vi "CVT1IndexWriteTest.vi"() -> (3 "Unit Test Framework Results":T1)   [LabVIEW 2013, in "UnitTests.lvlib"]
uses:
  UnitTests.lvlib
  <vilib>/utf/common/utf_test_result_troll.ctl
  <vilib>/utf/common/utf_test_result.ctl
  <vilib>/utf/common/utf_test_result_failure.ctl
  <vilib>/utf/common/utf_test_comparison_operators.ctl
  <vilib>/utf/common/utf_vi_tag.ctl
  <vilib>/NI/Current Value Table/Write Index.vi
  <vilib>/NI/Current Value Table/DataTypes/I32_Write Index.vi
  <vilib>/NI/Current Value Table/Read Index.vi
  <vilib>/NI/Current Value Table/DataTypes/I32_Read Index.vi
  <vilib>/NI/Current Value Table/Compatibility/TagConverter.vi
  <vilib>/NI/Current Value Table/Create Tags.vi
  <vilib>/NI/Current Value Table/Memory Block.vi
  <vilib>/NI/Current Value Table/DataTypes/I32_Memory Block.vi
  <vilib>/utf/NI_UnitTestFramework.lvlib
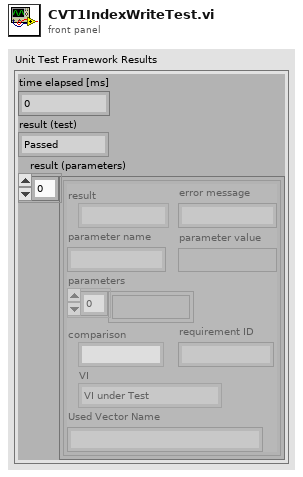
[diagram p1: front panel]
types:
  T1 = typedef "NI_UnitTestFramework.lvlib/utf_test_result_troll.ctl" = cluster{"time elapsed [ms]":u32, "result (test)":T2, "result (parameters)":T3[]}
  T2 = typedef "NI_UnitTestFramework.lvlib/utf_test_result.ctl" = enum16{"Passed", "Failed", "Error", "Skipped", "Not Processed"}
  T3 = typedef "NI_UnitTestFramework.lvlib/utf_test_result_failure.ctl" = cluster{"result":T2, "error message":string, "parameter name":string, "parameter value":variant, "parameters":variant[], "comparison":T4, "requirement ID":string, "VI":T5, "Used Vector Name":string}
  T4 = typedef "NI_UnitTestFramework.lvlib/utf_test_comparison_operators.ctl" = enum16{"=", "!=", ">", ">=", "<", "<=", "range", "symmetric tolerance", "asymmetric tolerance", "string contains", "string not contain", "array size", "string length", "array range", "by element", "array range (limit array)", "user-defined", "array contains", "array not contain", "vector length", "= (elm)", "!= (elm)", "= (case insensitive)", "!= (case insensitive)"}
  T5 = typedef "NI_UnitTestFramework.lvlib/utf_vi_tag.ctl" = enum16{"Setup VI", "VI under Test", "Teardown VI"}
  T6 = typedef "cvt_Tag Configuration.ctl" = cluster{"Name":string, "Data Type":T7, "Array":bool, "Size":u32, "Default":string, "Enum":string[], "Description":string}
  T7 = typedef "cvt_Data Types.ctl" = enum16{"Bool", "U8", "I32", "Double", "String", "Enum"}
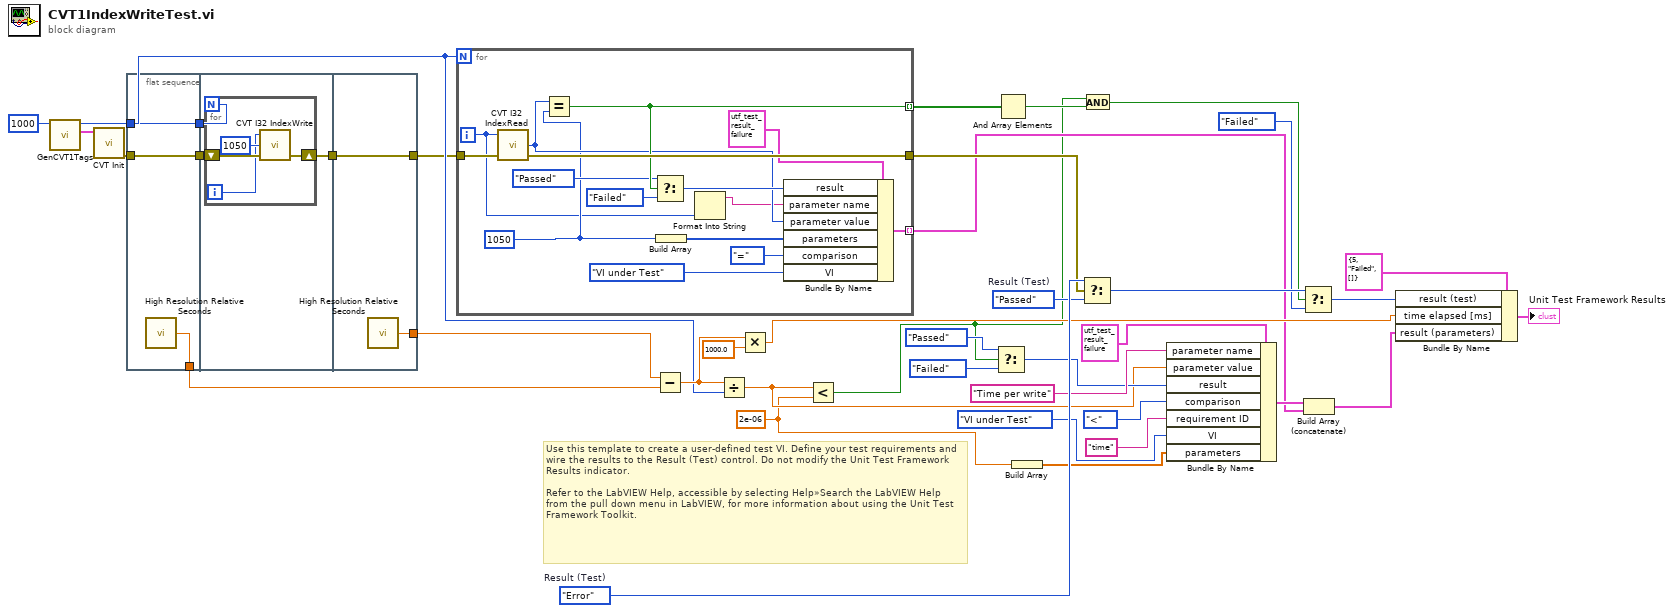
[diagram p0: block diagram]
diagram:
  w5 = 2e-06 ("y")
  w34 = utf_test_result."Error"  # Result (Test)
  w33 = utf_test_result."Passed"  # Result (Test)
  # "Use this template to create a user-defined test VI. Define your test requirements and wire the results to the Result (Test) control. Do not modify the Unit Test Framework Results indicator. \n\nRefer to the LabVIEW Help, accessible by selecting Help»Search the LabVIEW Help from the pull down menu in LabVIEW, for more information about using the Unit Test Framework Toolkit."
  n1 = call "GenCVT1Tags.vi"("Number of Tags in"=1000) -> ("Tags"=w27:T6[], "Number of Tags out"=w20:i32)  [unwired: 8 in, 1 out]
  n2 = call <vilib>:"CVT Init.vi"("Tag List"=w27) -> ("error out"=w26:errorcluster)  [unwired: 10 in]
  n3 = flat-sequence {
    tunnel: [w42] -> w36
    tunnel: w26 -> [w40]
    tunnel: [w41] -> w25
    tunnel: w20 -> [w41]
    tunnel: [w40] -> w24
    tunnel: w25 -> [w45]
    tunnel: w24 -> [w44]
    tunnel: [w43] -> w23
    tunnel: [w51] -> w37
    tunnel: w23 -> [w50]
    tunnel: [w50] -> w19
    frame #0 {
      n4 = call <vilib>:"High Resolution Relative Seconds.vi"() -> ("relative seconds"=w42:dbl)
    }
    frame #1 {
      n5 = for {
        N: w45 -> [_]
        shift-right: [w48] -> w43
        shift-left: w44 -> [w49]
        i -> [w46]
        n6 = call <vilib>:"CVT I32 IndexWrite.vi"("error in (no error)"=w49, "Value"=1050, "Tag Index"=w46) -> ("error out"=w48:errorcluster)  [unwired: 2 in]
      }
    }
    frame #2 {
      n7 = call <vilib>:"High Resolution Relative Seconds.vi"() -> ("relative seconds"=w51:dbl)
    }
  }
  n8 = for {
    N: w20 -> [_]
    tunnel: w19 -> [w66]
    tunnel: [w65] -> w18
    tunnel: [w62] -> w17 mode=indexing
    tunnel: [w58] -> w3 mode=indexing
    i -> [w53]
    w54 = 1050 ("Value")
    n9 = call <vilib>:"CVT I32 IndexRead.vi"("error in (no error)"=w66, "Tag Index"=w53) -> ("error out"=w65:errorcluster, "Value"=w55:i32)  [unwired: 2 in]
    n10 = Equal?(x=w55, y=w54) -> (x = y?=w62:bool)
    n11 = Select(t=utf_test_result."Passed" ("result"), s=w62, f=utf_test_result."Failed" ("result")) -> (s? t:f=w59:T2)
    n12 = Build Array(w54) -> (w56:i32[])
    n13 = Format Into String(w53) -> (resulting string=w52:string)  [unwired: 3 in, 1 out]
    n14 = Bundle By Name(cluster=T3 {"result"=enum."Passed", "error message"="", "parameter name"="", "parameter value"=variant, "parameters"=[], "comparison"=enum."=", "requirement ID"="", "VI"=enum."Setup VI", "Used Vector Name"=""} ("Unit Test Framework - result (parameters)"), "result"=w59, "parameter name"=w52, "parameter value"=w55, "parameters"=w56, "comparison"=utf_test_comparison_operators."=", "VI"=utf_vi_tag."VI under Test") -> (w58:T3)
  }
  n15 = Subtract(x=w37, y=w36) -> (x-y=w22:dbl)
  n16 = Divide(x=w22, y=w20) -> (x/y=w8:dbl)
  n17 = Multiply(x=w22, y=1000.0) -> (x*y=w28:dbl)
  n18 = Less?(x=w8, y=w5) -> (x < y?=w1:bool)
  n19 = Select(t=utf_test_result."Passed" ("result"), s=w1, f=utf_test_result."Failed" ("result")) -> (s? t:f=w9:T2)
  n20 = And Array Elements(Boolean array=w17) -> (logical AND=w16:bool)
  n21 = Build Array(w5) -> (w4:dbl[])
  n22 = Select(t=w34, s=w18, f=w33) -> (s? t:f=w15:T2)
  n23 = And(x=w1, y=w16) -> (x .and. y?=w2:bool)
  n24 = Bundle By Name(cluster=T3 {"result"=enum."Passed", "error message"="", "parameter name"="", "parameter value"=variant, "parameters"=[], "comparison"=enum."=", "requirement ID"="", "VI"=enum."Setup VI", "Used Vector Name"=""} ("Unit Test Framework - result (parameters)"), "parameter name"="Time per write", "parameter value"=w8, "result"=w9, "comparison"=utf_test_comparison_operators."<", "requirement ID"="time", "VI"=utf_vi_tag."VI under Test", "parameters"=w4) -> (w31:T3)
  n25 = Select(t=w15, s=w2, f=utf_test_result."Failed") -> (s? t:f=w13:T2)
  n26 = Build Array (concatenate)(w31, w3) -> (w30:T3[])
  n27 = Bundle By Name(cluster=T1 {"time elapsed [ms]"=5, "result (test)"=enum."Failed", "result (parameters)"=[]} ("Unit Test Framework - Result"), "result (test)"=w13, "time elapsed [ms]"=w28, "result (parameters)"=w30) -> (→"Unit Test Framework Results":T1)
